vi "RespiratoryControl.vi"(10 "Output Rate (ms)":u32=10 min=6 max=100000 step=1) -> ()   [LabVIEW 2019]
doc: "This VI is designed to output a sine wave with a DC offset of 2.5V and is especially intended for the USB-6008 and USB-6009. These devices are unique in the fact that they only support software timed analog output and their output range is 0V to 5V."
uses:
  <vilib>/Utility/error.llb/DialogType.ctl
  <vilib>/ptbypt/NI_PtbyPt.lvlib
panel:
  out "Output Data 2":dbl(graph)
  in  "Expiration Pause":dbl
  in  "Expiration Flow":dbl
  in  "Inspiration Pause":dbl=25.0
  in  "Inspiration Flow":dbl=50.0
  in  "Exhalation Flow Percent":dbl=0.25 min=0.25 max=0.75
  in  "Inhalation Flow Percent":dbl=0.4 min=0.25 max=0.75
  in  "Inhalation Percent":dbl=0.25 min=0.25 max=0.75 step=0.1
  # "Timing Parameters"
  # "Pressure Parameters"
  # "Waveform Parameters"
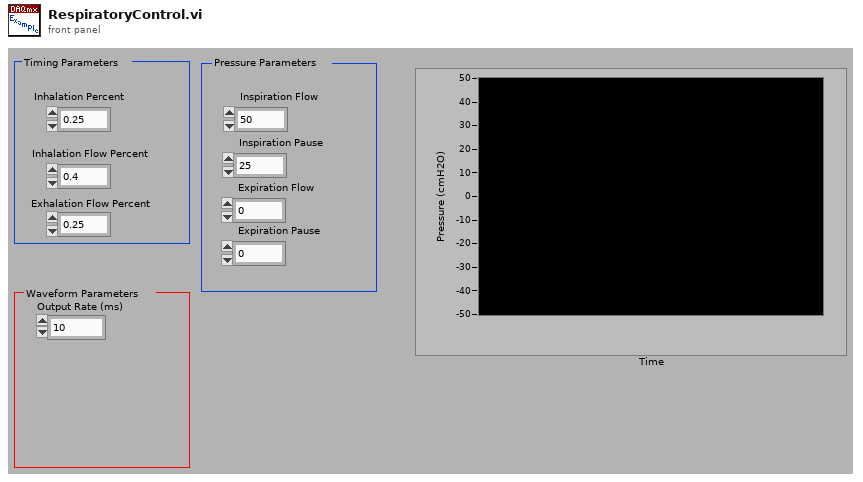
[diagram p1: front panel]
types:
  T1 = typedef "DialogType.ctl" = u16
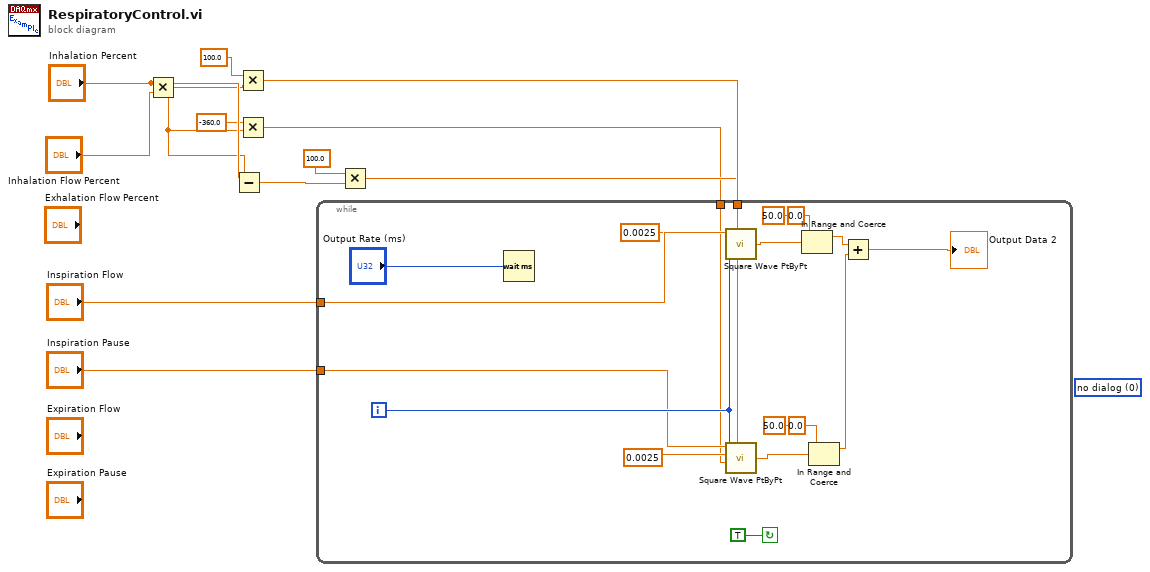
[diagram p0: block diagram]
diagram:
  (unwired) T1 0 items=["no dialog", "OK message", "continue or stop message", "OK message + warnings", "continue/stop + warnings"] ("type of dialog (OK msg:1)")
  n1 = Multiply(x="Inhalation Percent", y="Inhalation Flow Percent") -> (x*y=w3:dbl)
  n2 = Subtract(x="Inhalation Percent", y=w3) -> (x-y=w6:dbl)
  n3 = Multiply(x=100.0, y=w3) -> (x*y=w8:dbl)
  n4 = Multiply(x=-360.0, y=w3) -> (x*y=w1:dbl)
  n5 = Multiply(x=100.0, y=w6) -> (x*y=w4:dbl)
  n6 = while {
    tunnel: "Inspiration Flow" -> [w29]
    tunnel: "Inspiration Pause" -> [w25]
    tunnel: w8 -> [w23]
    tunnel: w4 -> [w22]
    tunnel: w1 -> [w21]
    i -> [w26]
    stop <- TRUE continue-if-true
    n7 = Wait (ms)(milliseconds to wait="Output Rate (ms)") -> ()  [unwired: 1 out]
    n8 = call <vilib>:"Square Wave PtByPt.vi"("amplitude"=w29, "frequency"=0.0025, "time"=w26, "duty cycle (%)"=w23) -> ("square wave"=w20:dbl)  [unwired: 1 in]
    n9 = call <vilib>:"Square Wave PtByPt.vi"("amplitude"=w25, "frequency"=0.0025, "phase"=w21, "time"=w26, "duty cycle (%)"=w22) -> ("square wave"=w18:dbl)
    n10 = In Range and Coerce(upper limit=50.0, x=w20, lower limit=0.0) -> (coerced(x)=w17:dbl)  [unwired: 1 out]
    n11 = In Range and Coerce(upper limit=50.0, x=w18, lower limit=0.0) -> (coerced(x)=w16:dbl)  [unwired: 1 out]
    n12 = Add(x=w17, y=w16) -> (x+y=→"Output Data 2":dbl)
  }
